vi "Generate SysDef Path.vi"() -> (0 "System Definition path":path)   [LabVIEW 2019, in "FPGA Addon DMA Channel Unit Tests.lvclass"]
uses:
  FPGA Addon DMA Channel Unit Tests.lvclass
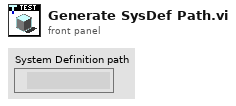
[diagram p1: front panel]
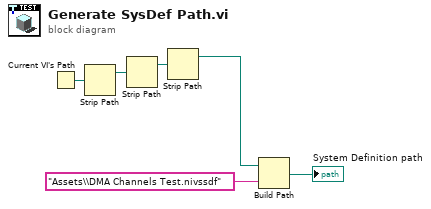
[diagram p0: block diagram]
diagram:
  n1 = Current VI's Path() -> (path=w6:path)
  n2 = Strip Path(path=w6) -> (stripped path=w5:path)  [unwired: 1 out]
  n3 = Strip Path(path=w5) -> (stripped path=w4:path)  [unwired: 1 out]
  n4 = Strip Path(path=w4) -> (stripped path=w3:path)  [unwired: 1 out]
  n5 = Build Path(base path=w3, name or relative path="Assets\\DMA Channels Test.nivssdf") -> (appended path=→"System Definition path":path)
